vi "StoredKey.vi"(9 "HMAC parameters":T1={"Salt"="salt123", "Iterations"=4096}, 10 "Un-hashed client Key":string, 11 "Secret":string="secret") -> (3 "StoredKey":u8[](array[numeric]))   [LabVIEW 2020, in "wamplv.lvlib" / "WampScramAuthenticator.lvclass"]
uses:
  WampScramAuthenticator.lvclass
  TypeDefs/HMAC parameters.ctl
  WampScramAuthenticator.lvclass/WampScramAuthenticator.ctl
  HashLib/HashLib.lvclass
  Utils/Utils.lvclass
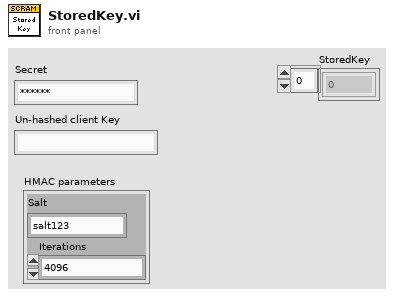
[diagram p1: front panel]
types:
  T1 = typedef "wamplv.lvlib/WampScramAuthenticator.lvclass/HMAC parameters.ctl" = cluster{"Salt":string, "Iterations":i32}
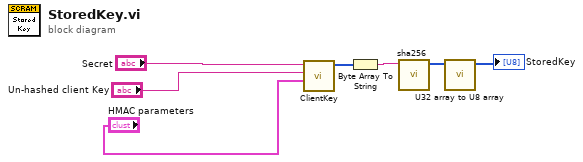
[diagram p0: block diagram]
diagram:
  n1 = call "ClientKey.vi"("HMAC parameters"="HMAC parameters", "Un-hashed client Key"="Un-hashed client Key", "Secret"="Secret") -> ("ClientKey"=w4:u8[])  [unwired: 8 in]
  n2 = Byte Array To String(unsigned byte array=w4) -> (string=w6:string)
  n3 = call "sha256.vi"("data"=w6) -> ("sha256"=w5:u32[])  [unwired: 10 in]
  n4 = call "U32 array to U8 array.vi"("Array in"=w5) -> ("Array out"=→"StoredKey":u8[])  [unwired: 10 in]
